vi "lr_step.vi"(0 "L_R":enum16{"r", "l"}(ring), 1 "Delay":i32, 2 "D":dbl, 3 "Step":i32) -> ()   [LabVIEW 2017]
uses:
  Constant.vi
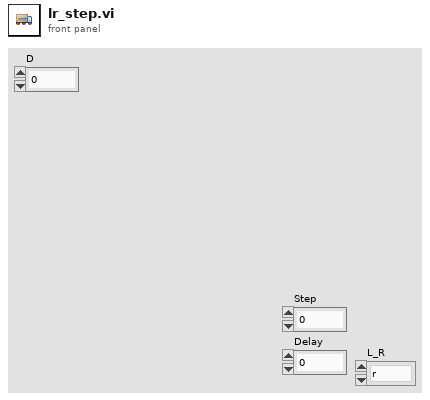
[diagram p1: front panel]
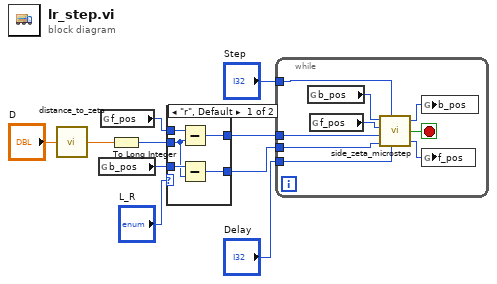
[diagram p0: block diagram]
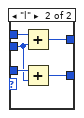
[diagram p2: hidden frame]
diagram:
  n1 = call "distance_to_zeta.vi"("D"="D") -> ("wheel_zeta"=w6:dbl)
  n2 = global read "Constant.vi" "b_pos"() -> (w8:i32)
  n3 = global read "Constant.vi" "f_pos"() -> (w7:i32)
  n4 = To Long Integer(number=w6) -> (32bit integer=w5:i32)
  n5 = case shown="\"r\", Default" "L_R" {
    tunnel: w8 -> [w15 w20]
    tunnel: w7 -> [w14 w19]
    tunnel: w5 -> [w13 w18]
    tunnel: [w12 w17] -> w4
    tunnel: [w11 w16] -> w3
    frame "r", Default {
      n6 = Subtract(x=w14, y=w13) -> (x-y=w11:i32)
      n7 = Subtract(x=w15, y=w13) -> (x-y=w12:i32)
    }
    frame "l" {
      n8 = Add(x=w19, y=w18) -> (x+y=w16:i32)
      n9 = Add(x=w20, y=w18) -> (x+y=w17:i32)
    }
  }
  n10 = while {
    tunnel: "Step" -> [w29]
    tunnel: "Delay" -> [w28]
    tunnel: w4 -> [w22]
    tunnel: w3 -> [w21]
    stop <- w27 stop-if-true
    n11 = global read "Constant.vi" "b_pos"() -> (w23:i32)
    n12 = global read "Constant.vi" "f_pos"() -> (w24:i32)
    n13 = call "side_zeta_microstep.vi"("Zeta_B"=w23, "Step"=w29, "Zeta_F"=w24, "taget_f"=w21, "Delay"=w28, "target_b"=w22) -> ("OZeta_b"=w26:i32, "Done"=w27:bool, "Ozeta_f"=w25:i32)
    n14 = global write "Constant.vi" "b_pos"(w26) -> ()
    n15 = global write "Constant.vi" "f_pos"(w25) -> ()
  }
